vi "Update System Log.vi"(8 "error in":errorcluster, 11 "Message":string) -> (0 "error out":errorcluster)   [LabVIEW 2018, in "Testing UI 1.lvlib"]
doc: "This subVI enqueues the named action in to the communications queue along with the input data."
uses:
  Testing UI 1.lvlib
  Private Controls/Module Action.ctl
  Private Controls/Module Data.ctl
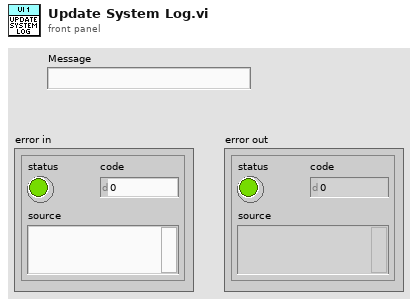
[diagram p1: front panel]
types:
  T1 = typedef "Testing UI 1.lvlib/Module Action.ctl" = enum8{"Init", "Open FP", "Timeout", "New Report Value", "Update Test Info", "Record Data", "Update Report Path", "SetFuelPressure", "Error", "Exit", "Update System Log", "Load APU Setup Data", "Threshold ALERT", "Engine Start Val Change", "Value to Record"}
  T2 = typedef "Testing UI 1.lvlib/Module Data.ctl" = cluster{"Data":variant, "Action":T1}
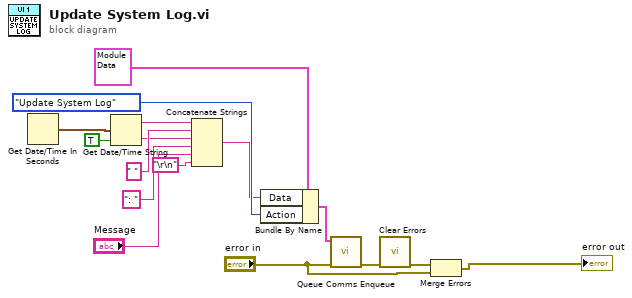
[diagram p0: block diagram]
diagram:
  n1 = Get Date/Time In Seconds() -> (seconds since 1Jan1904=w5:timestamp)
  n2 = Get Date/Time String(seconds (now)=w5, want seconds? (F)=TRUE) -> (date string=w10:string, time string=w12:string)  [unwired: 1 in]
  n3 = Concatenate Strings(w10, " " ("string"), w12, ": " ("string"), "Message", "\r\n") -> (w7:string)
  n4 = Bundle By Name(cluster=T2 {"Data"=variant, "Action"=enum."Init"} ("element"), "Data"=w7, "Action"=Module_Action."Update System Log") -> (w16:T2)
  n5 = call "Queue Comms Enqueue.vi"("error in (no error)"="error in", "element"=w16) -> ("error out"=w4:errorcluster)  [unwired: 9 in]
  n6 = call <vilib>:"Clear Errors.vi"("error in (no error)"=w4) -> ("error out"=w1:errorcluster)  [unwired: 5 in, 1 out]
  n7 = Merge Errors(w1, "error in") -> (→"error out":errorcluster)
